vi "Processing Step.vi"(8 "error in (no error)":errorcluster, 11 "Caching in":refnum<class "Caching.lvclass">) -> (0 "error out":errorcluster, 2 "Step":T1[](array[typedef]), 3 "Caching out":refnum<class "Caching.lvclass">)   [LabVIEW 2020, in "HTTP Server.lvlib" / "Caching.lvclass"]
uses:
  Caching.lvclass
  Processing Step.ctl
  HTTP Server.lvlib
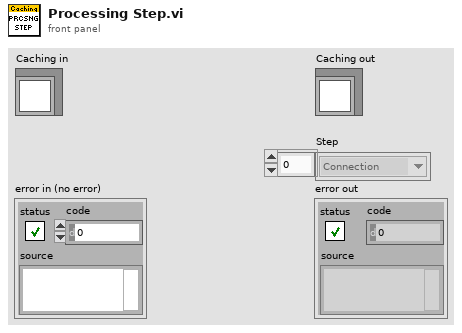
[diagram p1: front panel]
types:
  T1 = typedef "HTTP Server.lvlib/Processing Step.ctl" = enum16{"Connection", "Request", "Routing", "Controller Init", "Controller", "Response", "Complete", "Exception"}
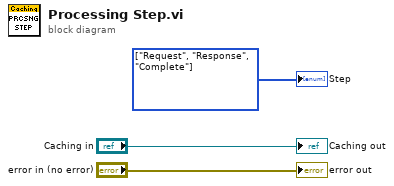
[diagram p0: block diagram]
diagram:
  w1 = T1[] [enum."Request", enum."Response", enum."Complete"] items=["Connection", "Request", "Routing", "Controller Init", "Controller", "Response", "Complete", "Exception"] ("Step")
  "error out" <- "error in (no error)"
  "Caching out" <- "Caching in"
  "Step" <- w1
